vi "Python Email.vi"(0 "Path to Python.exe":path=path "C:/Program Files/Python310/python.exe", 7 "To:":string, 9 "Subject:":string="Swoish Grain Control ALARM", 11 "Message:":string) -> (4 "Raw Python String Output":string="successfully sent the mail\r\n", 6 "Converted Output":i32, 8 "Return Code":i32, 10 "Standard Error":string, 15 "error out":errorcluster)   [LabVIEW 2020]
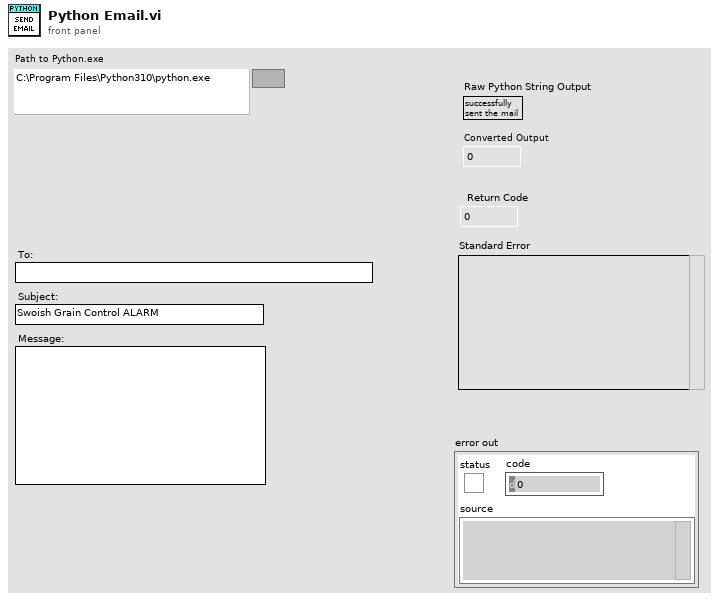
[diagram p1: front panel]
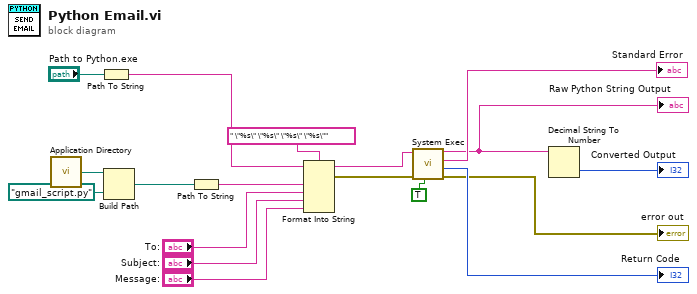
[diagram p0: block diagram]
diagram:
  n1 = call <vilib>:"Application Directory.vi"() -> ("Application Directory"=w3:path)
  n2 = Path To String(path="Path to Python.exe") -> (string=w11:string)
  n3 = Build Path(base path=w3, name or relative path=path "gmail_script.py") -> (appended path=w1:path)
  n4 = Path To String(path=w1) -> (string=w15:string)
  n5 = Format Into String(format string=" \"%s\" \"%s\" \"%s\" \"%s\"", initial string=w11, w15, "To:", "Subject:", "Message:") -> (resulting string=w14:string, error out=w12:errorcluster)  [unwired: 1 in]
  n6 = call <vilib>:"System Exec.vi"("run minimized? (F)"=TRUE, "error in (no error)"=w12, "command line"=w14) -> ("error out"=→"error out":errorcluster, "return code"=→"Return Code":i32, "standard error"=→"Standard Error":string, "standard output"=w9:string)  [unwired: 5 in]
  "Raw Python String Output" <- w9
  n7 = Decimal String To Number(string=w9) -> (number=→"Converted Output":i32)  [unwired: 2 in, 1 out]
